vi "oax_gsWaterfall Plot.vi"() -> ()   [LabVIEW 2017]
doc: "This is Order Analysis Toolkit demo VI."
uses:
  <vilib>/addons/Sound and Vibration/Order Analysis/Tach Process/SoundVib_TachProcess.lvlib
  <vilib>/Waveform/WDTOps.llb/WDT Waveform Duration DBL.vi
  <vilib>/addons/Sound and Vibration/Order Analysis/Resample Order Tracking/SoundVib_OrderTracking.lvlib
  <vilib>/addons/Sound and Vibration/Order Analysis/Data Presentation/SoundVib_SpectralDisplay.lvlib
  <vilib>/addons/_XControls/Waterfall Graph/SVX Waterfall Graph.xctl
panel:
  out "Waterfall Plot":T1(xcontrol) caption="Waterfall Graph"
  in  "windows info":cluster{"window type":u32, "window length":i32}={"window type"=62, "window length"=2048} {"window length" min=2; "window type" items=["None"=0, "Hanning"=1, "Hamming"=2, "Blackman-Harris"=3, "Exact Blackman"=4, "Blackman"=5, "Flat Top"=6, "4 Term B-Harris"=7, "7 Term B-Harris"=8, "Low Sidelobe"=9, "Gaussian"=62]}
  in  "Select Data":i32(listbox)
  in  "STOP":bool
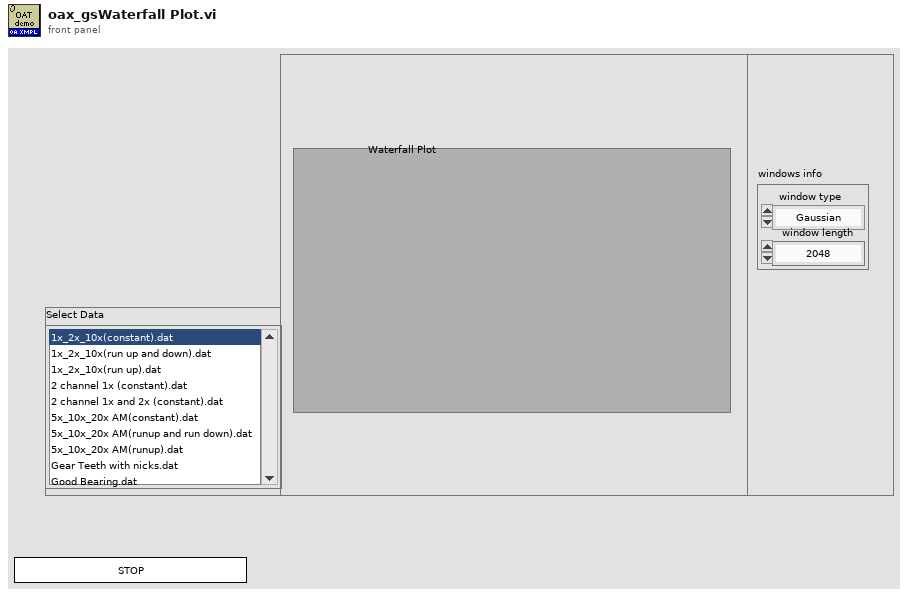
[diagram p1: front panel]
types:
  T1 = cluster{"z0":dbl, "dz":dbl, "Plots":cluster{"x0":dbl, "dx":dbl, "Y":dbl[]}[]}
  T2 = enum16{"Frequency-Time", "Time-Frequency", "Order-Time", "Time-Order"}
  T3 = typedef "SoundVib_TachProcess.lvlib/speed profile.ctl" = cluster{"time [s]":dbl[], "speed [RPM]":dbl[]}
  T4 = cluster{"z0":dbl, "dz":dbl, "waveforms":cluster{"f0":dbl, "df":dbl, "magnitude":dbl[]}[]}
  T5 = cluster{"x-axis unit label":string, "y-axis unit label":string, "z-axis unit label":string}
  T6 = cluster{"z0":dbl, "dz":dbl, "plots":cluster{"x0":dbl, "dx":dbl, "Y":dbl[]}[]}
  T7 = cluster{"pulse / rev":i32, "threshold (auto)":dbl, "slope (Rising)":u16}
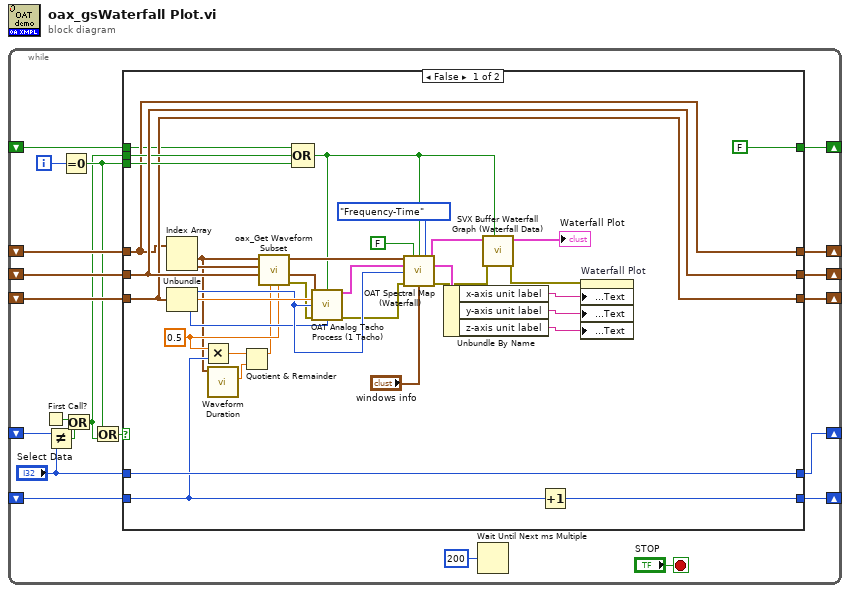
[diagram p0: block diagram]
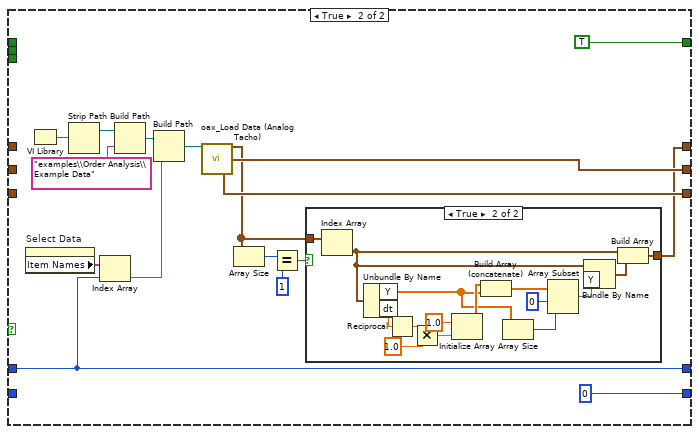
[diagram p2: hidden frame]
diagram:
  n1 = while {
    shift-right: [w17] -> _
    shift-left: _ -> [w18]
    shift-right: [w15] -> _
    shift-left: _ -> [w21]
    shift-right: [w14] -> _
    shift-left: _ -> [w19]
    shift-right: [w13] -> _
    shift-left: _ -> [w12]
    shift-right: [w3] -> _
    shift-left: _ -> [w4]
    shift-right: [w2] -> _
    shift-left: _ -> [w1]
    i -> [w11]
    stop <- "STOP" stop-if-true
    n2 = First Call?() -> (First Call?: T/F=w7:bool)
    n3 = Not Equal?(x=w18, y="Select Data") -> (x != y?=w6:bool)
    n4 = Equal To 0?(x=w11) -> (x = 0?=w10:bool)
    n5 = Or(x=w7, y=w6) -> (x .or. y?=w5:bool)
    n6 = Or(x=w10, y=w5) -> (x .or. y?=w9:bool)
    n7 = case shown="False" w9 {
      tunnel: w21 -> [w38 _]
      tunnel: w19 -> [w55 _]
      tunnel: [w56 w73] -> w17
      tunnel: "Select Data" -> [w56 w73]
      tunnel: [w38 w58] -> w15
      tunnel: [w55 w71] -> w14
      tunnel: [w49 w70] -> w13
      tunnel: w12 -> [w49 _]
      tunnel: w5 -> [w53 _]
      tunnel: w10 -> [w52 _]
      tunnel: w4 -> [w43 _]
      tunnel: [w45 0] -> w3
      tunnel: [FALSE TRUE] -> w2
      tunnel: w1 -> [w34 _]
      frame False {
        w44 = 0.5 ("y")
        n8 = Index Array(array=w38) -> (element #1=w42:waveform(dbl), element #2=w50:waveform(dbl))  [unwired: 2 in]
        n9 = Unbundle(w49) -> ("pulse / rev"=w47:i32, "threshold (auto)"=w48:dbl, "slope (Rising)"=w46:u16)
        n10 = Multiply(x=w44, y=w43) -> (x*y=w40:dbl)
        n11 = call-poly <vilib>:"Waveform Duration.vi"("waveform in"=w42) -> ("duration"=w41:dbl)  [unwired: 8 in, 2 out]
        n12 = Quotient & Remainder(x=w40, y=w41) -> (x-y*floor(x/y)=w39:dbl)  [unwired: 1 out]
        n13 = call <vilib>:"oax_Get Waveform Subset.vi"("duration"=w44, "start index"=w39, "Tach Signal"=w55, "Vibration Signal Y"=w50, "Vibration Signal X"=w42) -> ("error out"=w33:errorcluster, "Tach Signal out"=w54:waveform(dbl), "Vibration Signal X out"=w51:waveform(dbl))  [unwired: 3 in, 1 out]
        n14 = Compound Arithmetic op=OR(w34, w53, w52) -> (w24:bool)
        n15 = call <vilib>:"OAT Analog Tacho Process (1 Tacho).vi"("analog tacho signal"=w54, "reset? (F)"=w24, "threshold (auto)"=w48, "pulse/revolution (1)"=w47, "error in (no error)"=w33, "slope (Rising)"=w46) -> ("speed profile"=w57:T3, "error out"=w32:errorcluster)  [unwired: 5 in, 3 out]
        n16 = call <vilib>:"OAT Spectral Map (Waterfall).vi"("scaled signal [EU]"=w51, "dB on? (F)"=FALSE ("dB on (F)"), "reset? (F)"=w24, "plot type"=T2."Frequency-Time", "speed profile"=w57, "pulse/revolution (1)"=w47, "error in (no error)"=w32, "windows info"="windows info") -> ("waterfall graph"=w26:T4, "waterfall unit labels"=w31:T5, "error out"=w23:errorcluster)  [unwired: 3 in, 2 out]
        n17 = Unbundle By Name(w31) -> ("x-axis unit label"=w30:string, "y-axis unit label"=w29:string, "z-axis unit label"=w28:string)
        n18 = call <vilib>:"SVX Buffer Waterfall Graph (Waterfall Data).vi"("reset? (F)"=w24, "error in (no error)"=w23, "waterfall graph data"=w26) -> ("error out"=w22:errorcluster, "waterfall graph data out"=→"Waterfall Plot":T6)  [unwired: 7 in]
        n19 = Increment(x=w43) -> (x+1=w45:i32)
        n20 = property on="Waterfall Plot"(error in=w22, "XScale.NameLbl.Text"=w30, "YScale.NameLbl.Text"=w29, "ZScale.NameLbl.Text"=w28) -> ()  [unwired: 1 in, 2 out]
      }
      frame True {
        n21 = property on="Select Data" class="LstBox (strict)"() -> ("Item Names"=w74:string[])  [unwired: 2 in, 2 out]
        n22 = VI Library() -> (path=w66:path)
        n23 = Strip Path(path=w66) -> (stripped path=w65:path)  [unwired: 1 out]
        n24 = Index Array(array=w74, index=w73) -> (element=w68:string)
        n25 = Build Path(base path=w65, name or relative path="examples\\Order Analysis\\Example Data") -> (appended path=w69:path)
        n26 = Build Path(base path=w69, name or relative path=w68) -> (appended path=w67:path)
        n27 = call <vilib>:"oax_Load Data (Analog Tacho).vi"("Data Path In"=w67) -> ("vibration data"=w59:waveform(dbl)[], "analog tacho signal"=w71:waveform(dbl), "tacho info"=w70:T7)  [unwired: 8 in, 4 out]
        n28 = Array Size(array=w59) -> (size(s)=w62:i32)
        n29 = Equal?(x=w62, y=1) -> (x = y?=w60:bool)
        n30 = case shown="True" w60 {
          tunnel: w59 -> [w75 w90]
          tunnel: [w75 w89] -> w58
          frame False {
          }
          frame True {
            n31 = Index Array(array=w90) -> (element=w88:waveform(dbl))  [unwired: 1 in]
            n32 = Unbundle By Name(w88) -> ("Y"=w77:dbl[], "dt"=w86:dbl)
            n33 = Reciprocal(x=w86) -> (1/x=w85:dbl)
            n34 = Multiply(x=w85, y=1.0) -> (x*y=w83:dbl)
            n35 = Initialize Array(1.0 ("element"), w83) -> (w79:dbl[])
            n36 = Build Array (concatenate)(w79, w77) -> (w81:dbl[])
            n37 = Array Size(array=w77) -> (size(s)=w78:i32)
            n38 = Array Subset(array=w81, index=0, length=w78) -> (w76:dbl[])
            n39 = Bundle By Name(cluster=w88, "Y"=w76) -> (w87:waveform(dbl))
            n40 = Build Array(w88, w87) -> (w89:waveform(dbl)[])
          }
        }
      }
    }
    n41 = Wait Until Next ms Multiple(millisecond multiple=u32 200) -> ()  [unwired: 1 out]
  }
